vi "SimpleCaseStructurewithBoolean.vi"() -> ()   [LabVIEW 2019]
panel:
  in  "Boolean":bool
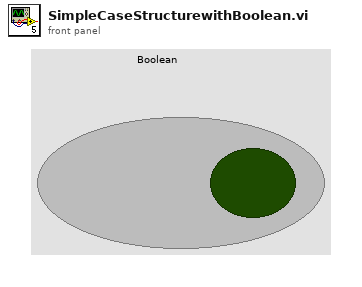
[diagram p1: front panel]
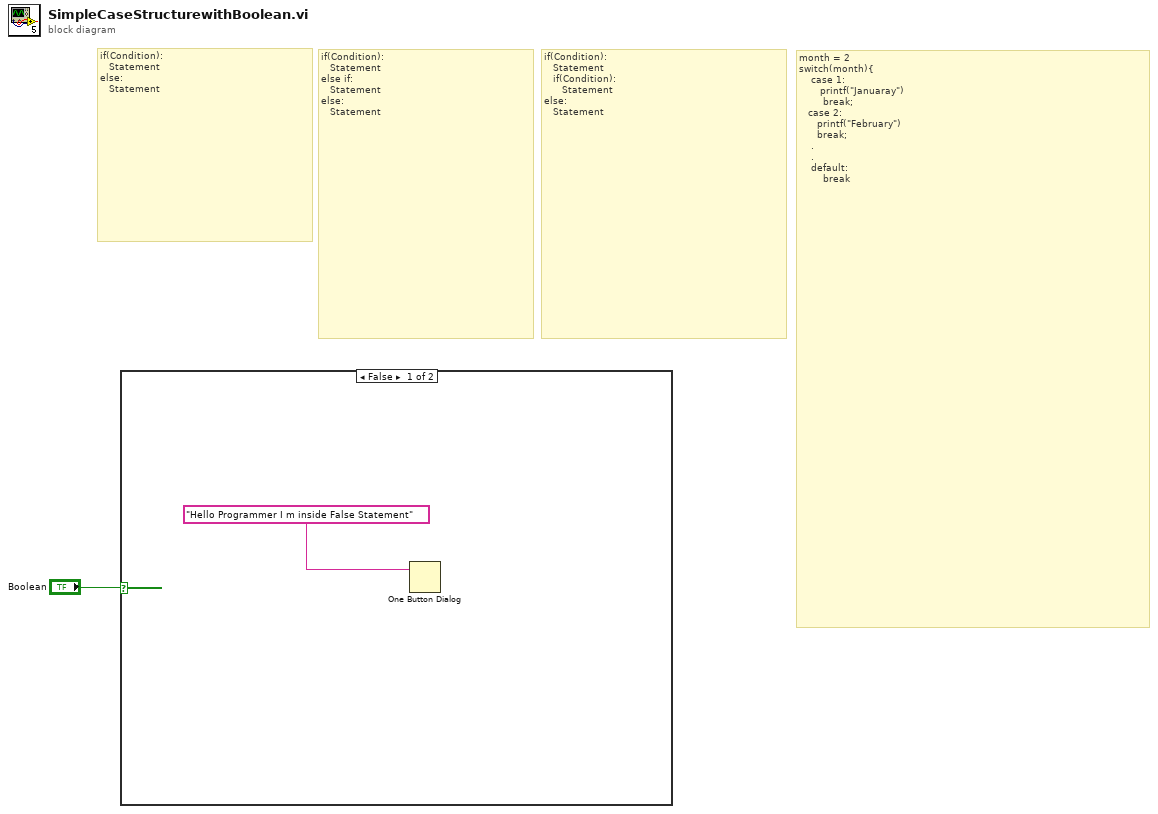
[diagram p0: block diagram]
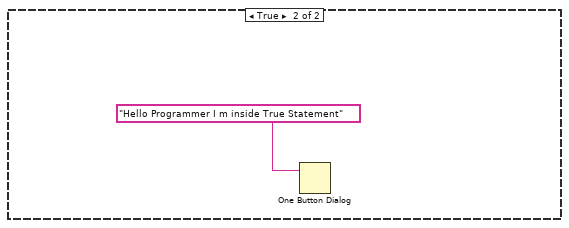
[diagram p2: hidden frame]
diagram:
  # "month = 2\nswitch(month){\n    case 1:\n       printf(\"Januaray\")\n        break;\n   case 2:\n      printf(\"February\")\n      break;\n    . \n    .\n    default:\n        break"
  # "if(Condition):\n   Statement\n   if(Condition):\n      Statement\nelse:\n   Statement"
  # "if(Condition):\n   Statement\nelse if:\n   Statement\nelse:\n   Statement"
  # "if(Condition):\n   Statement\nelse:\n   Statement"
  n1 = case shown="False" "Boolean" {
    frame False {
      n2 = One Button Dialog(message="Hello Programmer I m inside False Statement") -> ()  [unwired: 1 in, 1 out]
    }
    frame True {
      n3 = One Button Dialog(message="Hello Programmer I m inside True Statement") -> ()  [unwired: 1 in, 1 out]
    }
  }
